vi "Acquire T1 Waveform.vi"(7 "sampling frequency":dbl=98816000.0 format="%.2p", 11 "error in":errorcluster) -> (4 "Waveform":waveform(dbl), 15 "error out":errorcluster)   [LabVIEW 2012]
panel:
  out "actual Mbps":dbl format="%.2f"
  in  "Line Code":string="11001101011110010110011010101000101001001001"
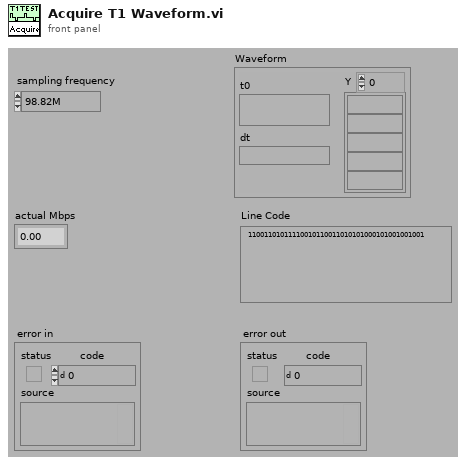
[diagram p1: front panel]
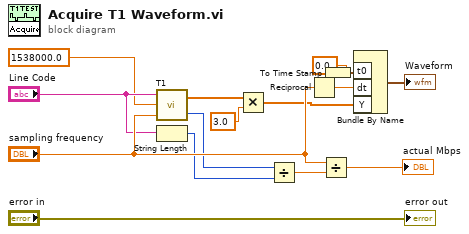
[diagram p0: block diagram]
diagram:
  n1 = call "T1.vi"("Sampling Frequency"="sampling frequency", "Frequency"=1538000.0 ("x"), "Line Code"="Line Code") -> ("NumberOfSamplesPerBit"=w11:i32, "Binary Waveform"=w4:dbl[])
  n2 = String Length(string="Line Code") -> (length=w10:i32)
  n3 = Multiply(x=w4, y=3.0) -> (x*y=w2:dbl[])
  n4 = Divide(x=w11, y=w10) -> (x/y=w9:dbl)
  n5 = Reciprocal(x="sampling frequency") -> (1/x=w7:dbl)
  n6 = Divide(x="sampling frequency", y=w9) -> (x/y=→"actual Mbps":dbl)
  n7 = To Time Stamp(1:0.0 ("t0")) -> (0:w1:timestamp)
  n8 = Bundle By Name("t0"=w1, "dt"=w7, "Y"=w2) -> (→"Waveform":waveform(dbl))  [unwired: 1 in]
  "error out" <- "error in"
